vi "关键参数组合 (子VI).vi"(9 "table":string="3090仪器参数", 10 "因子编码":string, 11 "DO":string[](array[string])) -> (3 "字符串":string)   [LabVIEW 2016, in "数据传输系统.lvlib"]
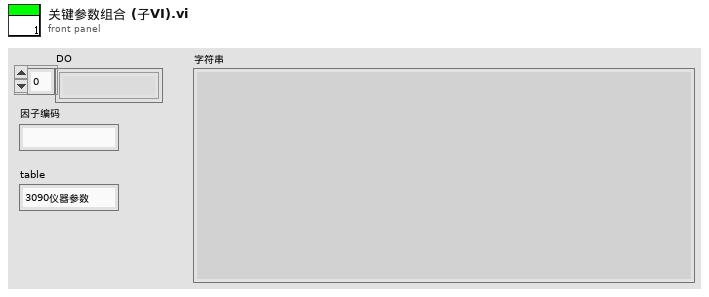
[diagram p1: front panel]
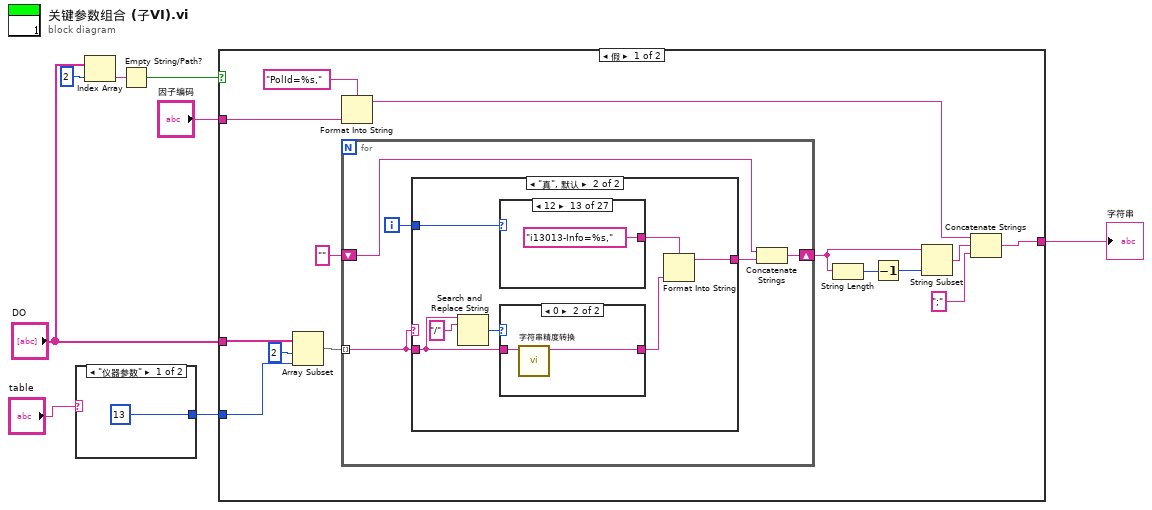
[diagram p0: block diagram]
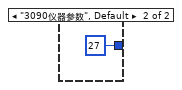
[diagram p2: hidden frame]
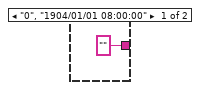
[diagram p3: hidden frame]
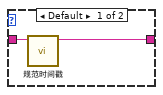
[diagram p4: hidden frame]
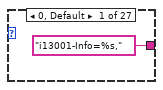
[diagram p5: hidden frame]
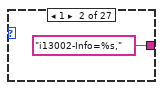
[diagram p6: hidden frame]
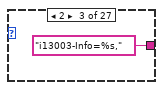
[diagram p7: hidden frame]
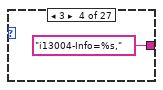
[diagram p8: hidden frame]
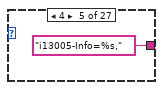
[diagram p9: hidden frame]
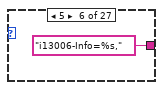
[diagram p10: hidden frame]
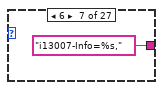
[diagram p11: hidden frame]
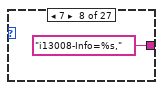
[diagram p12: hidden frame]
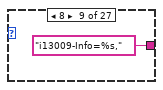
[diagram p13: hidden frame]
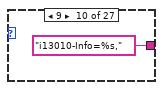
[diagram p14: hidden frame]
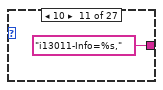
[diagram p15: hidden frame]
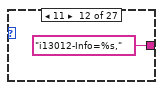
[diagram p16: hidden frame]
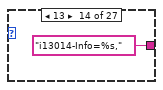
[diagram p17: hidden frame]
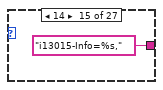
[diagram p18: hidden frame]
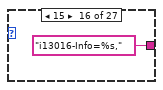
[diagram p19: hidden frame]
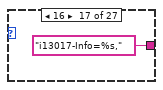
[diagram p20: hidden frame]
diagram:
  n1 = case shown="\"仪器参数\"" "table" {
    tunnel: [13 ("长度") 27 ("长度")] -> w1
    frame "仪器参数" {
    }
    frame "3090仪器参数", Default {
    }
  }
  n2 = Index Array(array="DO", index=2 ("索引")) -> (element=w7:string)
  n3 = Empty String/Path?(string/path=w7) -> (empty?=w6:bool)
  n4 = case shown="假" w6 {
    tunnel: [w23 ""] -> w5
    tunnel: "DO" -> [w22 _]
    tunnel: "因子编码" -> [w18 _]
    tunnel: w1 -> [w16 _]
    frame False {
      n5 = Array Subset(array=w22, index=2 ("索引"), length=w16) -> (w20:string[])
      n6 = Format Into String(format string="PolId=%s,", w18) -> (resulting string=w17:string)  [unwired: 2 in, 1 out]
      n7 = for {
        shift-right: [w26] -> w12
        shift-left: "" -> [w28]
        tunnel: w20 -> [w25] mode=indexing
        i -> [w29]
        n8 = case shown="\"真\", 默认" w25 {
          tunnel: w29 -> [_ w37]
          tunnel: ["" w35] -> w27
          tunnel: w25 -> [_ w32]
          frame "0", "1904/01/01 08:00:00" {
          }
          frame "真", Default {
            n9 = Search and Replace String(input string=w32, search string="/" ("搜索字符串")) -> (number of replacements=w34:i32)  [unwired: 6 in, 3 out]
            n10 = case shown="12" w37 {
              tunnel: ["i13001-Info=%s," "i13002-Info=%s," "i13003-Info=%s," "i13004-Info=%s," "i13005-Info=%s," "i13006-Info=%s," "i13007-Info=%s," "i13008-Info=%s," "i13009-Info=%s," "i13010-Info=%s," "i13011-Info=%s," "i13012-Info=%s," "i13013-Info=%s," "i13014-Info=%s," "i13015-Info=%s," "i13016-Info=%s," "i13017-Info=%s," "i13101-Info=%s," "i13102-Info=%s," "i13103-Info=%s," "i13104-Info=%s," "i13105-Info=%s," "i13106-Info=%s," "i13107-Info=%s," "i13108-Info=%s," "i13109-Info=%s," "i13110-Info=%s,"] -> w36
              frame 0, Default {
              }
              frame 1 {
              }
              frame 2 {
              }
              frame 3 {
              }
              frame 4 {
              }
              frame 5 {
              }
              frame 6 {
              }
              frame 7 {
              }
              frame 8 {
              }
              frame 9 {
              }
              frame 10 {
              }
              frame 11 {
              }
              frame 12 {
              }
              frame 13 {
              }
              frame 14 {
              }
              frame 15 {
              }
              frame 16 {
              }
              frame 17 {
              }
              frame 18 {
              }
              frame 19 {
              }
              frame 20 {
              }
              frame 21 {
              }
              frame 22 {
              }
              frame 23 {
              }
              frame 24 {
              }
              frame 25 {
              }
              frame 26 {
              }
            }
            n11 = case shown="0" w34 {
              tunnel: w32 -> [w39 w41]
              tunnel: [w38 w40] -> w31
              frame Default {
                n12 = call "规范时间戳.vi"("字符串"=w39) -> ("result string"=w38:string)  [unwired: 10 in]
              }
              frame 0 {
                n13 = call "字符串精度转换.vi"("输入字符串"=w41) -> ("输出字符串"=w40:string)  [unwired: 9 in, 1 out]
              }
            }
            n14 = Format Into String(format string=w36, w31) -> (resulting string=w35:string)  [unwired: 2 in, 1 out]
          }
        }
        n15 = Concatenate Strings(w28, w27) -> (w26:string)
      }
      n16 = String Length(string=w12) -> (length=w13:i32)
      n17 = Decrement(x=w13) -> (x-1=w14:i32)
      n18 = String Subset(string=w12, length (rest)=w14) -> (substring=w11:string)  [unwired: 1 in]
      n19 = Concatenate Strings(w17, w11, ";" ("字符串")) -> (w23:string)
    }
    frame True {
    }
  }
  "字符串" <- w5
